vi "Build Signals.vi"(5 "Controln":T1={"# scans"=0, "All"=FALSE, "Parameters of measurement"={"ODmin"=-0.35, "ODmax"=0.35, "Aq contol"=enum."fixed", "Wavelength_fix_index"=640, "WCM_limits"={"WCM_min"=0.0, "WCM_max"=0.0, "WCM_value"=0.0}, "WCM_corrections"=FALSE, "#cycles max"=5}}, 7 "WCM_values":sgl[](array[numeric]), 8 "error in (no error)":errorcluster, 9 "II channel seq":cluster{"BG":i32[], "Ie":i32[], "I0":i32[]}[](array[cluster]), 10 "I channel seq":cluster{"BG":i32[], "Ie":i32[], "I0":i32[]}[](array[cluster]), 11 "Detector in":refnum<class "Detector.lvclass">) -> (0 "error out":errorcluster, 1 "Signals so Send":T3, 2 "Signals":cluster{"wavelengths":dbl[], "Tableau":dbl[]}[](array[cluster]), 3 "Detector out":refnum<class "Detector.lvclass">, 4 "#PP":i32)   [LabVIEW 2015, in "Detector.lvclass"]
uses:
  Detector.lvclass
  dependecies/ControlsVIs/Clusters-def/Def_signals_from_DET.ctl
  dependecies/ControlsVIs/Clusters-def/Det-Read.ctl
  dependecies/ControlsVIs/Clusters-def/Parameters_measurement_def.ctl
  Detector.lvclass/Detector.ctl
  <vilib>/Analysis/baseanly.llb/Mean (DBL).vi
  dependecies/average-2Darray-SD_double.vi
  dependecies/average-2Darray-SD_int.vi
  <vilib>/Analysis/NI_AALBase.lvlib
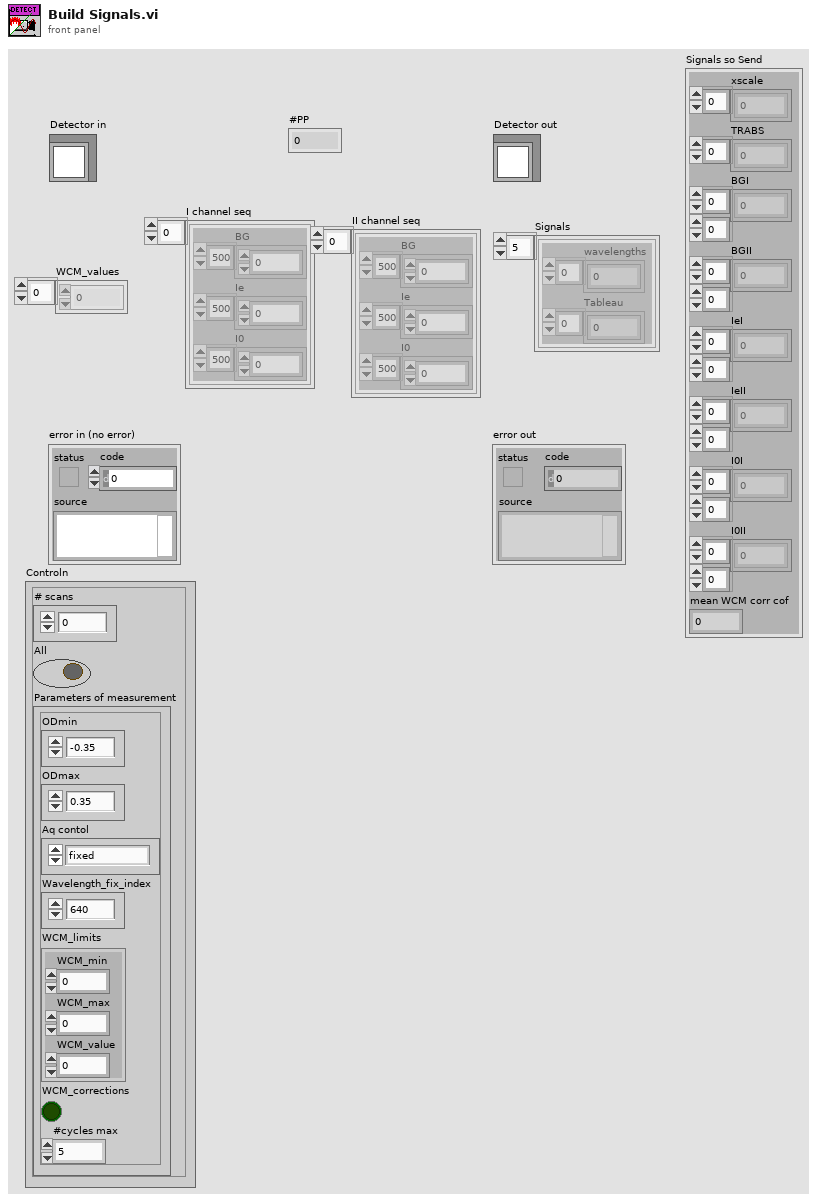
[diagram p1: front panel]
types:
  T1 = typedef "Detector.lvclass/Det-Read.ctl" = cluster{"# scans":i32, "All":bool, "Parameters of measurement":T2}
  T2 = typedef "Parameters_measurement_def.ctl" = cluster{"ODmin":dbl, "ODmax":dbl, "Aq contol":enum32{"fixed", "automatic", "fixed-auto"}, "Wavelength_fix_index":i32, "WCM_limits":cluster{"WCM_min":dbl, "WCM_max":dbl, "WCM_value":dbl}, "WCM_corrections":bool, "#cycles max":i32}
  T3 = typedef "Detector.lvclass/Def_signals_from_DET.ctl" = cluster{"xscale":sgl[], "TRABS":sgl[], "BGI":i32[][], "BGII":i32[][], "IeI":i32[][], "IeII":i32[][], "I0I":i32[][], "I0II":i32[][], "mean WCM corr cof":dbl}
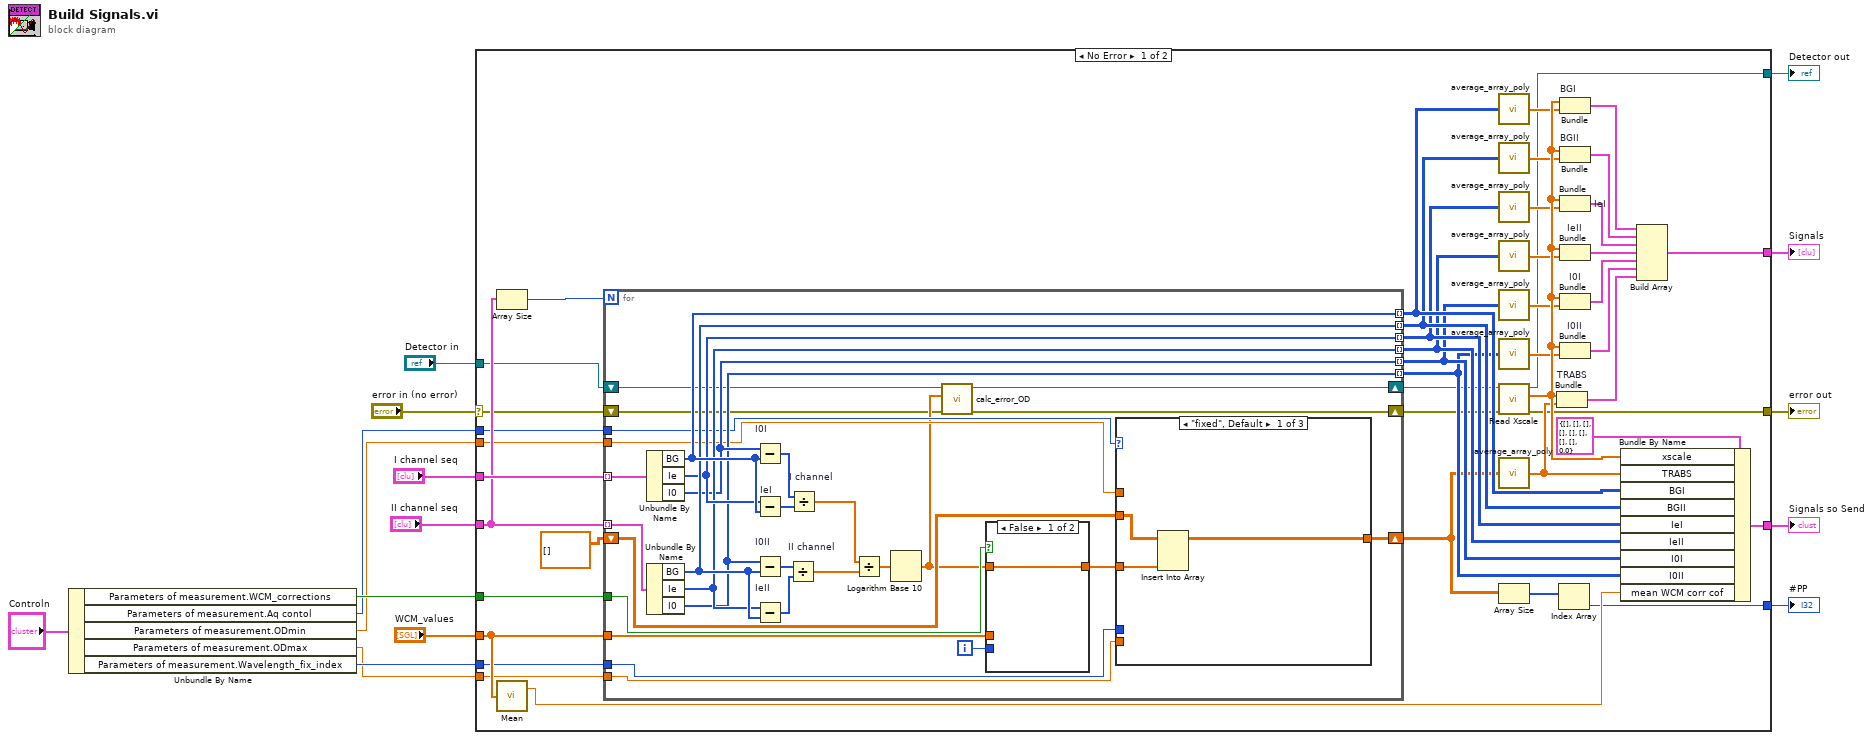
[diagram p0: block diagram]
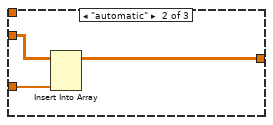
[diagram p2: hidden frame]
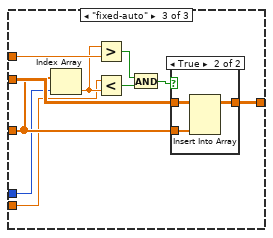
[diagram p3: hidden frame]
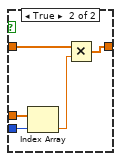
[diagram p5: hidden frame]
diagram:
  n1 = Unbundle By Name("Controln") -> ("Parameters of measurement.WCM_corrections"=w5:bool, "Parameters of measurement.Aq contol"=w4:enum32{"fixed", "automatic", "fixed-auto"}, "Parameters of measurement.ODmin"=w2:dbl, "Parameters of measurement.ODmax"=w1:dbl, "Parameters of measurement.Wavelength_fix_index"=w3:i32)
  n2 = case shown="No Error" "error in (no error)" {
    selector: "error in (no error)" -> [w20 w117]
    tunnel: [w22 w117] -> w14
    tunnel: [w21 w118] -> w15
    tunnel: "Detector in" -> [w19 w118]
    tunnel: [w53 _] -> w11
    tunnel: "WCM_values" -> [w38 _]
    tunnel: [w51 _] -> w9
    tunnel: "I channel seq" -> [w41 _]
    tunnel: "II channel seq" -> [w39 _]
    tunnel: w5 -> [w40 _]
    tunnel: [w23 _] -> w10
    tunnel: w4 -> [w29 _]
    tunnel: w3 -> [w28 _]
    tunnel: w2 -> [w27 _]
    tunnel: w1 -> [w26 _]
    frame No Error {
      n3 = Array Size(array=w39) -> (size(s)=w37:i32)
      n4 = call-poly <vilib>:"Mean.vi"("X"=w38) -> ("mean"=w50:dbl)  [unwired: 1 out]
      n5 = for {
        N: w37 -> [_]
        tunnel: w41 -> [w90] mode=indexing
        tunnel: w39 -> [w89] mode=indexing
        tunnel: [w82] -> w36 mode=indexing
        tunnel: [w81] -> w35 mode=indexing
        tunnel: w40 -> [w79]
        tunnel: w38 -> [w78]
        tunnel: [w76] -> w34 mode=indexing
        tunnel: [w75] -> w33 mode=indexing
        tunnel: [w74] -> w32 mode=indexing
        tunnel: [w73] -> w31 mode=indexing
        shift-right: [w71] -> w25
        shift-left: dbl[][] [] -> [w72]
        tunnel: w29 -> [w69]
        tunnel: w28 -> [w68]
        tunnel: w27 -> [w67]
        tunnel: w26 -> [w66]
        shift-right: [w63] -> w18
        shift-left: w19 -> [w64]
        shift-right: [w61] -> w17
        shift-left: w20 -> [w62]
        i -> [w77]
        n6 = Unbundle By Name(w90) -> ("BG"=w82:i32[], "Ie"=w76:i32[], "I0"=w74:i32[])
        n7 = Unbundle By Name(w89) -> ("BG"=w81:i32[], "Ie"=w75:i32[], "I0"=w73:i32[])
        n8 = Subtract "I0I"(x=w74, y=w82) -> (x-y=w83:i32[])
        n9 = Subtract "IeI"(x=w76, y=w82) -> (x-y=w80:i32[])
        n10 = Subtract "I0II"(x=w73, y=w81) -> (x-y=w84:i32[])
        n11 = Subtract "IeII"(x=w75, y=w81) -> (x-y=w85:i32[])
        n12 = Divide "II channel"(x=w84, y=w85) -> (x/y=w86:dbl[])
        n13 = Divide "I channel"(x=w83, y=w80) -> (x/y=w87:dbl[])
        n14 = Divide(x=w87, y=w86) -> (x/y=w88:dbl[])
        n15 = Logarithm Base 10(1:w88) -> (0:w65:dbl[])
        n16 = call "calc_error_OD.vi"("error in (no error)"=w62, "OD"=w65, "Detector in"=w64) -> ("error out"=w61:errorcluster, "Detector out"=w63:refnum<class "Detector.lvclass">)  [unwired: 7 in]
        n17 = case shown="False" w79 {
          tunnel: [w111 w115] -> w70
          tunnel: w65 -> [w111 w116]
          tunnel: w78 -> [_ w114]
          tunnel: w77 -> [_ w113]
          frame False {
          }
          frame True {
            n18 = Index Array(array=w114, index=w113) -> (element=w112:sgl)
            n19 = Multiply(x=w116, y=w112) -> (x*y=w115:dbl[])
          }
        }
        n20 = case shown="\"fixed\", Default" w69 {
          tunnel: w72 -> [w93 w96 w105]
          tunnel: [w92 w95 w106] -> w71
          tunnel: w70 -> [w91 w94 w104]
          tunnel: w68 -> [_ _ w103]
          tunnel: w67 -> [_ _ w102]
          tunnel: w66 -> [_ _ w100]
          frame "fixed", Default {
            n21 = Insert Into Array(array=w93, new element=w91) -> (w92:dbl[][])  [unwired: 2 in]
          }
          frame "automatic" {
            n22 = Insert Into Array(array=w96, new element=w94) -> (w95:dbl[][])  [unwired: 2 in]
          }
          frame "fixed-auto" {
            n23 = Index Array(array=w104, index=w103) -> (element=w101:dbl)
            n24 = Greater?(x=w101, y=w102) -> (0:w99:bool)
            n25 = Less?(x=w100, y=w101) -> (x < y?=w98:bool)
            n26 = And(x=w99, y=w98) -> (x .and. y?=w97:bool)
            n27 = case shown="True" w97 {
              tunnel: [w107 w110] -> w106
              tunnel: w105 -> [w107 w109]
              tunnel: w104 -> [_ w108]
              frame False {
              }
              frame True {
                n28 = Insert Into Array(array=w109, new element=w108) -> (w110:dbl[][])  [unwired: 2 in]
              }
            }
          }
        }
      }
      n29 = call-poly "average_array_poly.vi"("2D array"=w36) -> ("out array"=w47:dbl[])
      n30 = call-poly "average_array_poly.vi"("2D array"=w35) -> ("out array"=w46:dbl[])
      n31 = call-poly "average_array_poly.vi"("2D array"=w34) -> ("out array"=w45:dbl[])
      n32 = call-poly "average_array_poly.vi"("2D array"=w33) -> ("out array"=w44:dbl[])
      n33 = call-poly "average_array_poly.vi"("2D array"=w32) -> ("out array"=w43:dbl[])
      n34 = call-poly "average_array_poly.vi"("2D array"=w31) -> ("out array"=w42:dbl[])
      n35 = call "Read Xscale.vi"("error in (no error)"=w17, "Detector en entrée"=w18) -> ("error out"=w22:errorcluster, "Xscale"=w49:dbl[], "Detector en sortie"=w21:refnum<class "Detector.lvclass">)  [unwired: 7 in]
      n36 = call-poly "average_array_poly.vi"("2D array"=w25) -> ("out array"=w48:dbl[])
      n37 = Array Size(array=w25) -> (size(s)=w24:i32[])
      n38 = Bundle "TRABS"("Xscale"=w49, "out array"=w48) -> (w54:cluster{"Xscale":dbl[], "out array":dbl[]})  [unwired: 1 in]
      n39 = Index Array(array=w24) -> (element=w23:i32)  [unwired: 1 in]
      n40 = Bundle "BGI"("Xscale"=w49, "out array"=w47) -> (w59:cluster{"Xscale":dbl[], "out array":dbl[]})  [unwired: 1 in]
      n41 = Bundle "BGII"("Xscale"=w49, "out array"=w46) -> (w60:cluster{"Xscale":dbl[], "out array":dbl[]})  [unwired: 1 in]
      n42 = Bundle "IeI"("Xscale"=w49, "out array"=w45) -> (w58:cluster{"Xscale":dbl[], "out array":dbl[]})  [unwired: 1 in]
      n43 = Bundle "IeII"("Xscale"=w49, "out array"=w44) -> (w57:cluster{"Xscale":dbl[], "out array":dbl[]})  [unwired: 1 in]
      n44 = Bundle "I0I"("Xscale"=w49, "out array"=w43) -> (w56:cluster{"Xscale":dbl[], "out array":dbl[]})  [unwired: 1 in]
      n45 = Bundle "I0II"("Xscale"=w49, "out array"=w42) -> (w55:cluster{"Xscale":dbl[], "out array":dbl[]})  [unwired: 1 in]
      n46 = Bundle By Name(cluster=T3 {"xscale"=[], "TRABS"=[], "BGI"=[], "BGII"=[], "IeI"=[], "IeII"=[], "I0I"=[], "I0II"=[], "mean WCM corr cof"=0.0}, "xscale"=w49, "TRABS"=w48, "BGI"=w36, "BGII"=w35, "IeI"=w34, "IeII"=w33, "I0I"=w32, "I0II"=w31, "mean WCM corr cof"=w50) -> (w51:T3)
      n47 = Build Array(w59, w60, w58, w57, w56, w55, w54) -> (w53:cluster{"Xscale":dbl[], "out array":dbl[]}[])
    }
    frame Error {
    }
  }
  "error out" <- w14
  "Detector out" <- w15
  "Signals so Send" <- w9
  "Signals" <- w11
  "#PP" <- w10
